vi "DEV Set Power Level.vi"(10 "PowerLevel":i8, 11 "DevHandle":i32) -> (3 "function return":u8)   [LabVIEW 2010, in "usb_device.lvlib"]
doc: "unsigned char WINAPI DEV_SetPowerLevel(int DevHandle,char PowerLevel);"
uses:
  usb_device.lvlib
  USB2XXX/trunk/USB2XXX/USB2XXX/vs2019/Release/USB2XXX.dll
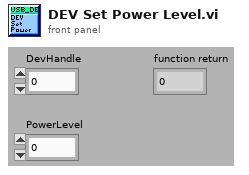
[diagram p1: front panel]
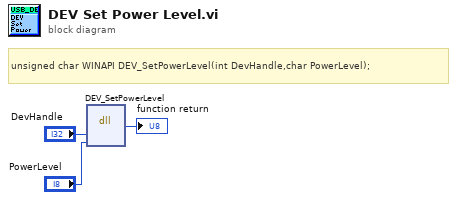
[diagram p0: block diagram]
diagram:
  # "unsigned char WINAPI DEV_SetPowerLevel(int DevHandle,char PowerLevel);"
  n1 = dll-call lib="E:/Projects/USB2XXX/trunk/USB2XXX/USB2XXX/vs2019/Release/USB2XXX.*" fn="DEV_SetPowerLevel"("DevHandle"="DevHandle", "PowerLevel"="PowerLevel") -> (→"function return":u8)  [unwired: 5 in, 2 out]
